vi "Output External.vi"(5 "Pulse Mode":i32(ring) items=["Pulse", "Clock"], 6 "Pulse Period":dbl, 7 "Polarity":i32(ring) items=["Negative", "Positive"], 8 "error in":errorcluster, 9 "Source":i32(ring) items=["Arm Event", "Trigger Event", "A Trigger", "B Trigger", "Capture Complete", "Operation Complete", "Master Summary Status Event", "Constant State", "Pulse Event", "Reference", "Limit Test Pass", "Probe Compensation"], 10 "State":i32(ring) items=["Active", "Inactive"], 11 "Instrument Handle In":i32) -> (0 "error out":errorcluster, 3 "Instrument Handle Out":i32)   [LabVIEW 8.6, in "ZTScopeM.lvlib"]
doc: "Configure the external output"
uses:
  ZTScopeM.lvlib
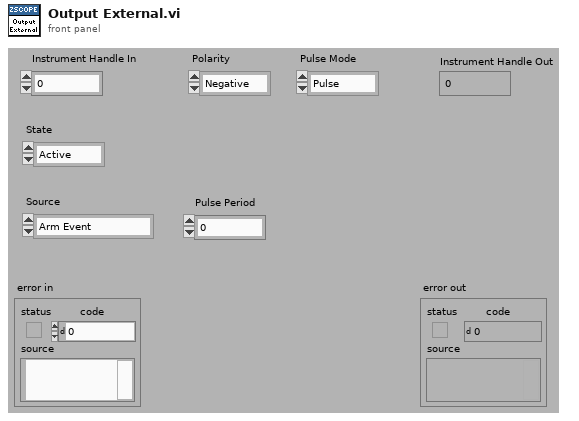
[diagram p1: front panel]
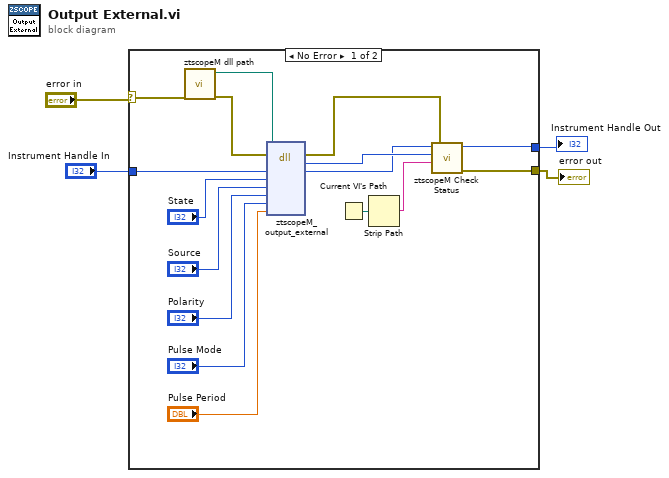
[diagram p0: block diagram]
diagram:
  n1 = case shown="No Error" "error in" {
    selector: "error in" -> [w8 w22]
    tunnel: [w10 w22] -> w1
    tunnel: "Instrument Handle In" -> [w20 w21]
    tunnel: [w9 w21] -> w3
    frame #0 {
      n2 = call "ztscopeM dll path.vi"("error in (no error)"=w8) -> ("error out"=w6:errorcluster, "<instrument>.dll path"=w7:path)  [unwired: 9 in]
      n3 = dll-call lib="C:/Program Files (x86)/National Instruments/LabVIEW 2013/instr.lib/ztscopem/ztscopeM.dll" fn="ztscopeM_output_external"(path in=w7, error in=w6, "instrumentHandle"=w20, "state"="State", "source"="Source", "polarity"="Polarity", "pulseMode"="Pulse Mode", "pulsePeriod"="Pulse Period") -> (error out=w5:errorcluster, w12:i32, "instrumentHandle"=w11:i32)  [unwired: 6 in, 1 out]
      n4 = Current VI's Path() -> (path=w14:path)
      n5 = Strip Path(path=w14) -> (name=w13:string)  [unwired: 1 out]
      n6 = call "ztscopeM Check Status.vi"("error in"=w5, "name of VI"=w13, "status (return code)"=w12, "instrument handle in"=w11) -> ("error out"=w10:errorcluster, "instrument handle out"=w9:i32)  [unwired: 2 in]
    }
    frame #1 {
    }
  }
  "Instrument Handle Out" <- w3
  "error out" <- w1
